vi "CheckStatus.vi"(11 "String IN":string) -> ()   [LabVIEW 2014]
panel:
  out "output cluster":T1
  in  "error IN":errorcluster
  out "error out":errorcluster
  out "Z":dbl
  out "Y":dbl
  out "X":dbl
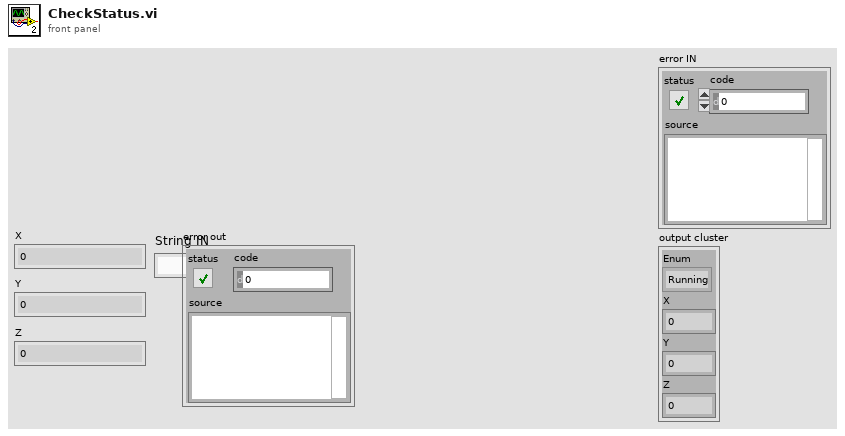
[diagram p1: front panel]
types:
  T1 = cluster{"Enum":enum16{"Running", "Waiting", "Pos", "IDLE"}, "X":dbl, "Y":dbl, "Z":dbl}
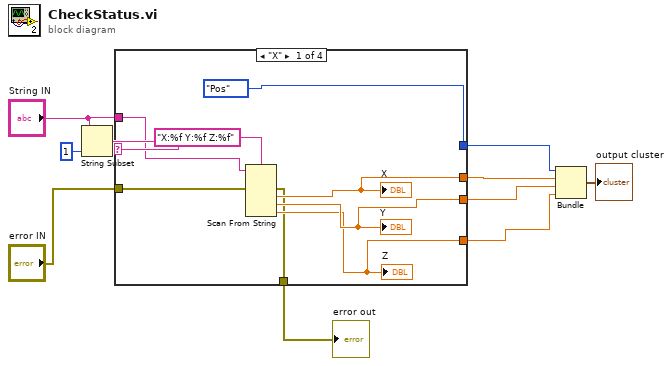
[diagram p0: block diagram]
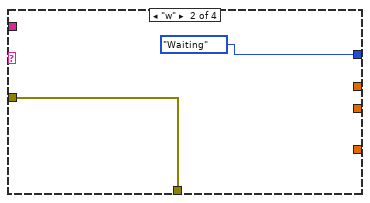
[diagram p2: hidden frame]
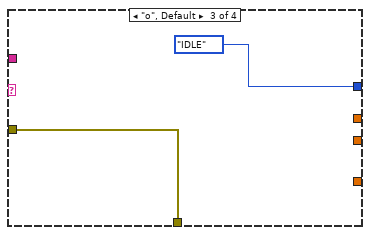
[diagram p3: hidden frame]
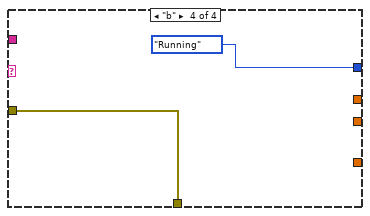
[diagram p4: hidden frame]
diagram:
  n1 = String Subset(string="String IN", length (rest)=1 ("length (rest)")) -> (substring=w9:string)  [unwired: 1 in]
  n2 = case shown="\"X\"" w9 {
    tunnel: [enum16{"Running", "Waiting", "Pos"}."Pos" ("Enum") enum16{"Running", "Waiting", "Pos"}."Waiting" ("Enum") enum16{"Running", "Waiting", "Pos", "IDLE"}."IDLE" ("Enum") enum16{"Running", "Waiting", "Pos"}."Running" ("Enum")] -> w7
    tunnel: "String IN" -> [w16 _ _ _]
    tunnel: [w15 _ _ _] -> w6
    tunnel: [w14 _ _ _] -> w5
    tunnel: [w13 _ _ _] -> w4
    tunnel: "error IN" -> [w12 w19 w21 w23]
    tunnel: [w11 w19 w21 w23] -> w2
    frame "X" {
      n3 = Scan From String(format string="X:%f Y:%f Z:%f", input string=w16, error in=w12) -> (error out=w11:errorcluster, output 1=w15:dbl, output 2=w14:dbl, output 3=w13:dbl)  [unwired: 4 in, 2 out]
      "X" <- w15
      "Y" <- w14
      "Z" <- w13
    }
    frame "w" {
    }
    frame "o", Default {
    }
    frame "b" {
    }
  }
  "error out" <- w2
  n4 = Bundle("Enum"=w7, "X"=w6, "Y"=w5, "Z"=w4) -> (→"output cluster":T1)  [unwired: 1 in]
